vi "Save ASCII Text to Unicode File.vi"() -> ()   [LabVIEW 2009]
panel:
  out "File Path":path
  out "File Contents (Hex)":string
  out "File Contents (Unicode Display)":string
  out "File Contents (ASCII Display)":string
  in  "String 2":string="World"
  in  "String 1":string="Hello"
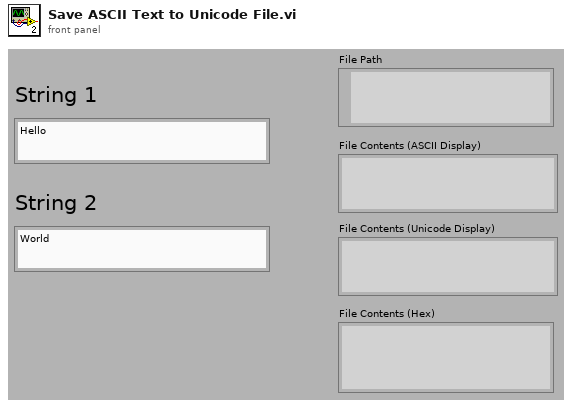
[diagram p1: front panel]
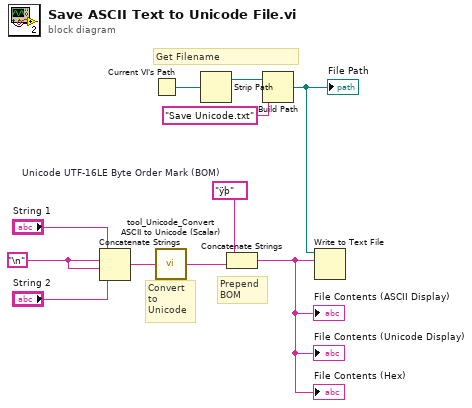
[diagram p0: block diagram]
diagram:
  w3 = "\n"
  w9 = "ÿþ"  # Unicode UTF-16LE Byte Order Mark (BOM)
  # "Convert to Unicode"
  # "Prepend BOM"
  # "Get Filename"
  n1 = Concatenate Strings("String 1", w3, w3, "String 2") -> (w2:string)
  n2 = Current VI's Path() -> (path=w7:path)
  n3 = call "tool_Unicode_Convert ASCII to Unicode (Scalar).vi"("ASCII"=w2) -> ("Unicode"=w1:string)  [unwired: 4 in]
  n4 = Strip Path(path=w7) -> (stripped path=w6:path)  [unwired: 1 out]
  n5 = Concatenate Strings(w9, w1) -> (w8:string)
  "File Contents (ASCII Display)" <- w8
  "File Contents (Unicode Display)" <- w8
  "File Contents (Hex)" <- w8
  n6 = Build Path(base path=w6, name or relative path="Save Unicode.txt") -> (appended path=w4:path)
  "File Path" <- w4
  n7 = Write to Text File(file (use dialog)=w4, text=w8) -> ()  [unwired: 2 in, 3 out]
